vi "lowPassFilter.vi"() -> ()   [LabVIEW 2020]
panel:
  out "Original":waveform(dbl)(graph)
  in  "Input Signal":path
  in  "Filter Select":u16(ring) items=["Lowpass", "Highpass", "Bandpass", "Bandstop", "Smoothing"]
  in  "Filter Order":i32(knob) scale=1.0..5.0
  in  "Filter Cut Off Frequency":dbl(knob) scale=1.0..20000.0
  out "Filtered Signal":dynamicdata(graph)
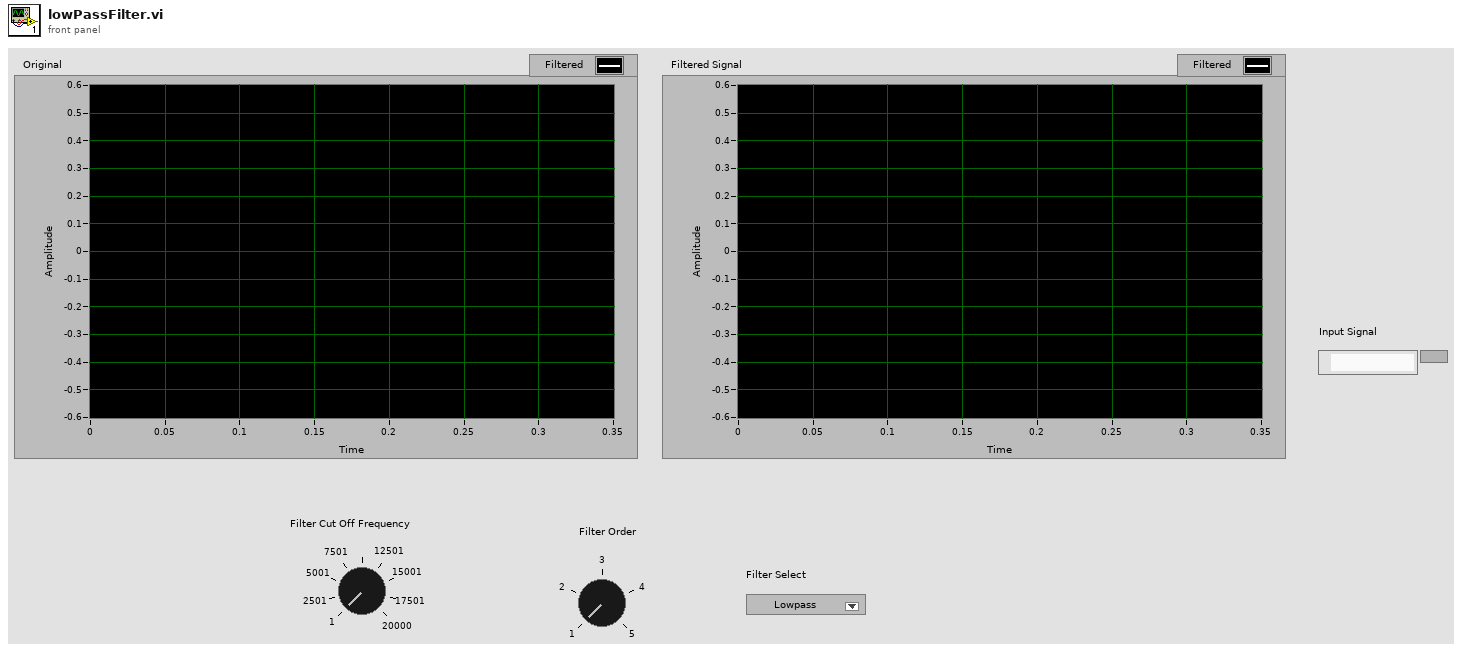
[diagram p1: front panel]
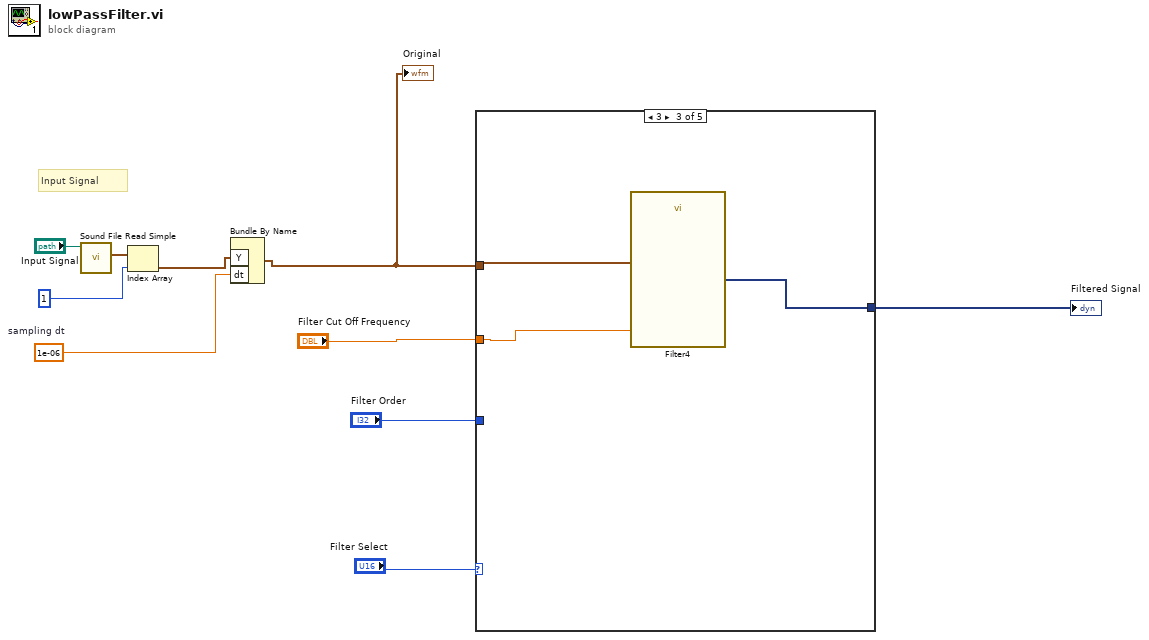
[diagram p0: block diagram]
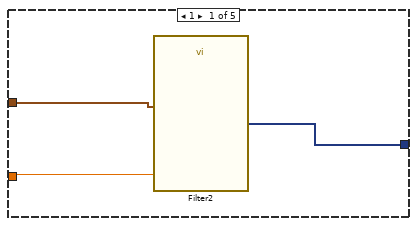
[diagram p2: hidden frame]
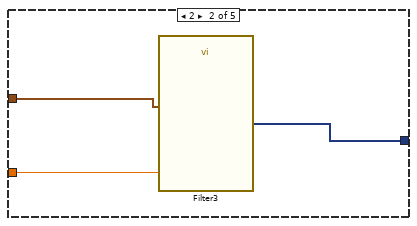
[diagram p3: hidden frame]
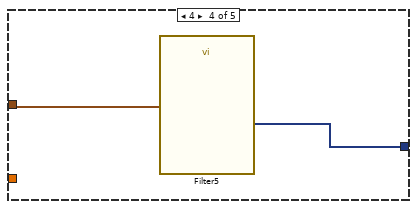
[diagram p4: hidden frame]
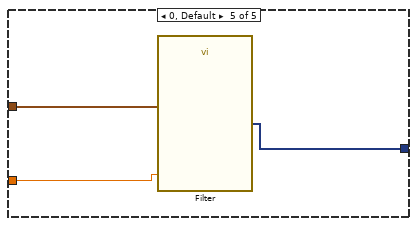
[diagram p5: hidden frame]
diagram:
  w2 = 1e-06  # sampling dt
  # "Input Signal"
  n1 = call <vilib>:"Sound File Read Simple.vi"("path"="Input Signal") -> ("data"=w5:waveform(dbl)[])  [unwired: 7 in, 3 out]
  n2 = Index Array(array=w5, index=1) -> (element=w3:waveform(dbl))
  n3 = Bundle By Name("Y"=w3, "dt"=w2) -> (w1:waveform(dbl))  [unwired: 1 in]
  "Original" <- w1
  n4 = case shown="3" "Filter Select" {
    tunnel: [w13 w16 w18 w21 w24] -> w10
    tunnel: "Filter Cut Off Frequency" -> [w12 w15 w19 _ w23]
    tunnel: "Filter Order" -> [_ _ _ _ _]
    tunnel: w1 -> [w11 w14 w17 w20 w22]
    frame 1 {
      n5 = call "Filter2"("Lower Cut-Off"=w12, "Signal"=w11) -> ("Filtered Signal"=w13:dynamicdata)  [unwired: 8 in, 1 out]
    }
    frame 2 {
      n6 = call "Filter3"("Lower Cut-Off"=w15, "Signal"=w14) -> ("Filtered Signal"=w16:dynamicdata)  [unwired: 8 in, 1 out]
    }
    frame 3 {
      n7 = call "Filter4"("Lower Cut-Off"=w19, "Signal"=w17) -> ("Filtered Signal"=w18:dynamicdata)  [unwired: 8 in, 1 out]
    }
    frame 4 {
      n8 = call "Filter5"("Signal"=w20) -> ("Filtered Signal"=w21:dynamicdata)  [unwired: 9 in, 1 out]
    }
    frame 0, Default {
      n9 = call "Filter"("Lower Cut-Off"=w23, "Signal"=w22) -> ("Filtered Signal"=w24:dynamicdata)  [unwired: 8 in, 1 out]
    }
  }
  "Filtered Signal" <- w10
